vi "Mittelwert vorgeben.vi"(11 "Komponente":u16(ring)) -> (3 "Mittelwert":sgl format="%.2f")   [LabVIEW 2020, in "EPA 1065.lvlib" / "Interference verificaton 1065-375.lvlib"]
uses:
  Interference verificaton 1065-375.lvlib
  Seiten/FT-IR/FGV FT-IR Aktionen.ctl
  Messdaten/Gewichtung (Stichprobe).ctl
  Messdaten/Aktionen FGV Messdaten.ctl
  Seiten/FT-IR/FT-IR.lvlib
  Messdaten/Messdaten.lvlib
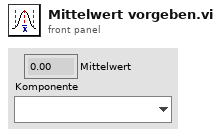
[diagram p1: front panel]
types:
  T1 = typedef "Messdaten.lvlib/Aktionen FGV Messdaten.ctl" = enum16{"lesen", "schreiben", "löschen", "Mittelwerte", "Komponente"}
  T2 = typedef "Messdaten.lvlib/Gewichtung (Stichprobe).ctl" = enum16{"Sample", "Population"}
  T3 = typedef "FT-IR.lvlib/FGV FT-IR Aktionen.ctl" = enum16{"lesen", "NOG setzen", "NOS setzen", "Initialisieren", "speichern", "ALLES setzen", "FT-IR Spektrum loggen", "Komm Stoppen", "Spektrum LogKonfig"}
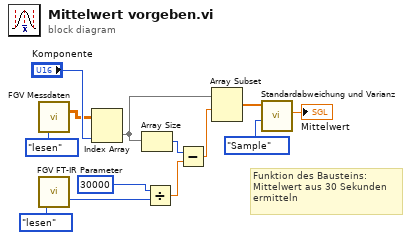
[diagram p0: block diagram]
diagram:
  # "Funktion des Bausteins:\nMittelwert aus 30 Sekunden \nermitteln"
  n1 = call "FGV Messdaten.vi"("Aktionen"=Aktionen_FGV_Messdaten."lesen") -> ("Messdaten"=w1:sgl[][])  [unwired: 6 in, 8 out]
  n2 = call "FGV FT-IR Parameter.vi"("Aktion"=FGV_FT-IR_Aktionen."lesen") -> ("Zykluszeit Messdatenverteiler"=w12:u32)  [unwired: 11 in, 7 out]
  n3 = Index Array(array=w1, index (col)="Komponente") -> (element=w2:sgl[])  [unwired: 1 in]
  n4 = Array Size(array=w2) -> (size(s)=w7:i32)
  n5 = Divide(x=30000, y=w12) -> (x/y=w6:dbl)
  n6 = Subtract(x=w7, y=w6) -> (x-y=w8:dbl)
  n7 = Array Subset(array=w2, index=w8) -> (w5:sgl[])  [unwired: 1 in]
  n8 = call "Standardabweichung und Varianz.vi"("Gewichtung (Stichprobe)"=Gewichtung_(Stichprobe)."Sample", "X"=w5) -> ("Mittelwert"=→"Mittelwert":sgl)  [unwired: 7 in, 2 out]
